vi "SyncMessage_CSM_CallerAndCallee.vi"(8 "error in (no error)":errorcluster, 10 "CSMCallee":string="CSMCallee", 11 "CSMCaller":string="CSMCaller") -> (0 "error out":errorcluster, 2 "Set API response out":string, 3 "Actual API Response out":string)   [LabVIEW 2017, in "testcase-SyncMessage.lvclass"]
uses:
  testcase-SyncMessage.lvclass
  src/user.lib/_NEVSTOP/Communicable State Machine(CSM)/Communicable State Machine.lvlib
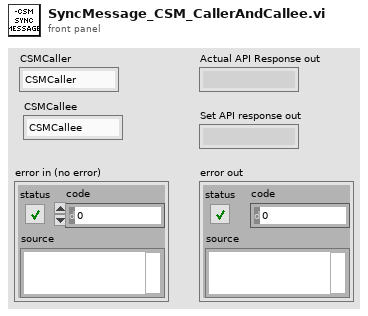
[diagram p1: front panel]
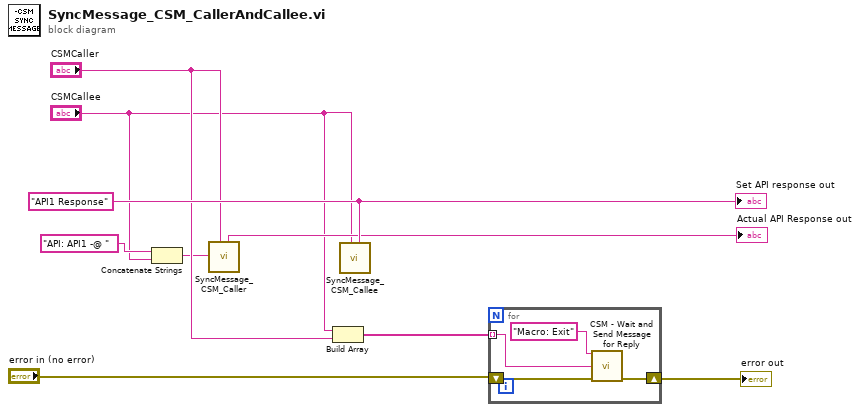
[diagram p0: block diagram]
diagram:
  w9 = "API1 Response" ("API response in")
  n1 = Concatenate Strings("API: API1 -@ " ("Intermodule Message in"), "CSMCallee") -> (w1:string)
  n2 = call "SyncMessage_CSM_Caller.vi"("Name (\"\" to Use UUID)"="CSMCaller", "Intermodule Message in"=w1) -> ("API received Response out"=→"Actual API Response out":string)  [unwired: 9 in]
  n3 = Build Array("CSMCallee", "CSMCaller") -> (w7:string[])
  n4 = call "SyncMessage_CSM_Callee.vi"("API response in"=w9, "Name (\"\" to Use UUID)"="CSMCallee") -> ()  [unwired: 10 in]
  n5 = for {
    shift-right: [w11] -> w8
    shift-left: "error in (no error)" -> [w12]
    tunnel: w7 -> [w10] mode=indexing
    n6 = call "CSM - Wait and Send Message for Reply.vi"("State"="Macro: Exit", "Target Module"=w10, "Error In (No Error)"=w12) -> ("error out"=w11:errorcluster)  [unwired: 10 in, 2 out]
  }
  "error out" <- w8
  "Set API response out" <- w9
